vi "stimulate_pose.vi"(4 "Injection point":T4, 6 "Stimulus":sgl[](array[numeric])=[0.0, 0.0, 0.0, 0.0, 0.0, 0.0] format="%#_3p", 8 "Pose in":T1, 10 "Parameters":T2={"Stimulus"={"Type"=enum."Off", "Phase"=0.0, "Amplitude"=[], "Injection point"=enum."Total pose", "Closed loop"=FALSE, "Offset"=[], "Tip -> world"=FALSE, "Frequency"=0.0, "Length"=0.0}, "Goal Filter A"={"Speedup max"=0.0, "Speedup thresh"=0.0, "Speedup nonlin"=0.0, "Filters"=[]}, "Mode controls"={"Hold"=FALSE, "Cancellation"=FALSE, "Goal filter"=FALSE, "Trigger"=FALSE}, "Manipulator type"=enum."Current piezo", "Manipulator calibration"={"Tool offsets"=[[0.0, 0.0, 36200.0]], "Handle light calibration"=[], "Base pivots"=[], "Output pivots"=[], "Length center"=0.0, "Workspace height"=[], "Workspace diameter"=[0.0, 0.0, 36200.0], "Stack travel"=400.0, "Saturation pos"=375.0, "Inverse filters"=[], "Strut length"=0.0}, "Network"={"Remote Host"="", "Send Status"=FALSE, "Send Port"=0, "Recv Commands"=FALSE, "Recv Port"=0}, "Goal Filter B"={"Speedup max"=0.0, "Speedup thresh"=0.0, "Speedup nonlin"=0.0, "Filters"=[]}, "Cancellation"={"KP"={"XY"=0.0, "Rxy"=0.0, "Z"=0.0, "Rz"=0.0}, "KI"=0.0, "KD"={"XY"=0.0, "Rxy"=0.0, "Z"=0.0, "Rz"=0.0}, "Max vel"=20.0, "Max acc"=0.001, "Int error limit"=3.0, "RCM gain"=0.0, "Bypass"=FALSE, "Degraded gain"=0.0}, "Transition time"=0.0, "Estimation"={"Link"={"Measure noise"=[], "Process noise"=[], "Alt process noise"=[], "Alt turnoff cycles"=20, "Innovation limit"=[], "Residue threshold"=0.0, "Enable"=FALSE}, "Handle"={"Measure noise"=[], "Process noise"=[], "State limits"=[], "Innovation limit"=[], "Prediction Lookahead"=0.0, "Enable"=FALSE}}} {"Transition time" format="%_3f"; "Cancellation"."Degraded gain" min=0 max=1 step=0.1 format="%#_3p"; "Cancellation"."RCM gain" min=0 max=1 step=0.1 format="%#_3p"; "Cancellation"."KD"."Rz" min=-1 max=1 step=0.01 format="%#_3p"; "Cancellation"."KD"."Rxy" min=-1 max=1 step=0.01 format="%#_3p"; "Cancellation"."KD"."Z" min=-1 max=1 step=0.01 format="%#_3p"; "Cancellation"."KD"."XY" min=-1 max=1 step=0.01 format="%#_3p"; "Cancellation"."KI" min=0 max=1 step=0.01 format="%#_3p"; "Cancellation"."KP"."Rz" min=-1 max=1 step=0.01 format="%#_3p"; "Cancellation"."KP"."Rxy" min=-1 max=1 step=0.01 format="%#_3p"; "Cancellation"."KP"."Z" min=-1 max=1 step=0.01 format="%#_3p"; "Cancellation"."KP"."XY" min=-1 max=1 step=0.01 format="%#_3p"; "Cancellation"."Max acc" format="%#_3p"; "Goal Filter B"."Filters"."V limit range" format="%_3p"; "Goal Filter B"."Filters"."V limit" format="%_3p"; "Goal Filter B"."Filters"."Upper Q" format="%_3f"; "Goal Filter B"."Filters"."Upper Fc" format="%_3p"; "Goal Filter B"."Filters"."Lower Q" format="%_3f"; "Goal Filter B"."Filters"."Scale factor" format="%_3f"; "Goal Filter B"."Filters"."Lower Fc" format="%_3p"; "Goal Filter B"."Speedup nonlin" format="%_3p"; "Goal Filter B"."Speedup thresh" format="%_3p"; "Goal Filter B"."Speedup max" format="%_3p"; "Manipulator calibration"."Strut length" format="%#_4p"; "Manipulator calibration"."Saturation pos" format="%#.1f"; "Manipulator calibration"."Stack travel" format="%#.1f"; "Manipulator calibration"."Length center" format="%#_4p"; "Manipulator calibration"."Output pivots" format="%#_6f"; "Manipulator calibration"."Base pivots" format="%#_6f"; "Manipulator calibration"."Handle light calibration" format="%#.1f"; "Goal Filter A"."Filters"."V limit range" format="%_3p"; "Goal Filter A"."Filters"."V limit" format="%_3p"; "Goal Filter A"."Filters"."Upper Q" format="%_3f"; "Goal Filter A"."Filters"."Upper Fc" format="%_3p"; "Goal Filter A"."Filters"."Lower Q" format="%_3f"; "Goal Filter A"."Filters"."Scale factor" format="%_3f"; "Goal Filter A"."Filters"."Lower Fc" format="%_3p"; "Goal Filter A"."Speedup nonlin" format="%_3p"; "Goal Filter A"."Speedup thresh" format="%_3p"; "Goal Filter A"."Speedup max" format="%_3p"; "Stimulus"."Length" min=0.0 max=100.0 step=100.0 format="%#_4p"; "Stimulus"."Frequency" min=0.0 step=100.0 format="%#_4g"; "Stimulus"."Offset" format="%#_3p"; "Stimulus"."Amplitude" format="%#_3p"; "Stimulus"."Phase" min=-180.0 max=360.0 step=100.0 format="%#.2f"}) -> (1 "Pose out":T1)   [LabVIEW 2014]
uses:
  <vilib>/Analysis/Matrix/Datatypes/RealMatrix.ctl
  injection_point.ctl
  Micron params.ctl
  stimulus.ctl
  filtering/goal_loop_parms.ctl
  mode_conrols.ctl
  manipulator_cal.ctl
  asap/labview/testing/probe_calibration.ctl
  host/network_params.ctl
  cancellation/sq_control_params.ctl
  cancellation/decoupled_gain.ctl
  cancellation/estimation_controls.ctl
  <vilib>/Analysis/baseanly.llb/Real A x B.vi
  initialization/micron_globals.vi
  <vilib>/Analysis/Matrix/Numeric/Conversions/Array To Matrix - RA2.vi
  <vilib>/Analysis/NI_AALBase.lvlib
  <vilib>/Analysis/Matrix/NI_Matrix.lvlib
panel:
  # "Inject stimulus to pose.  Stimulus is interpreted as XYZ and Euler angles."
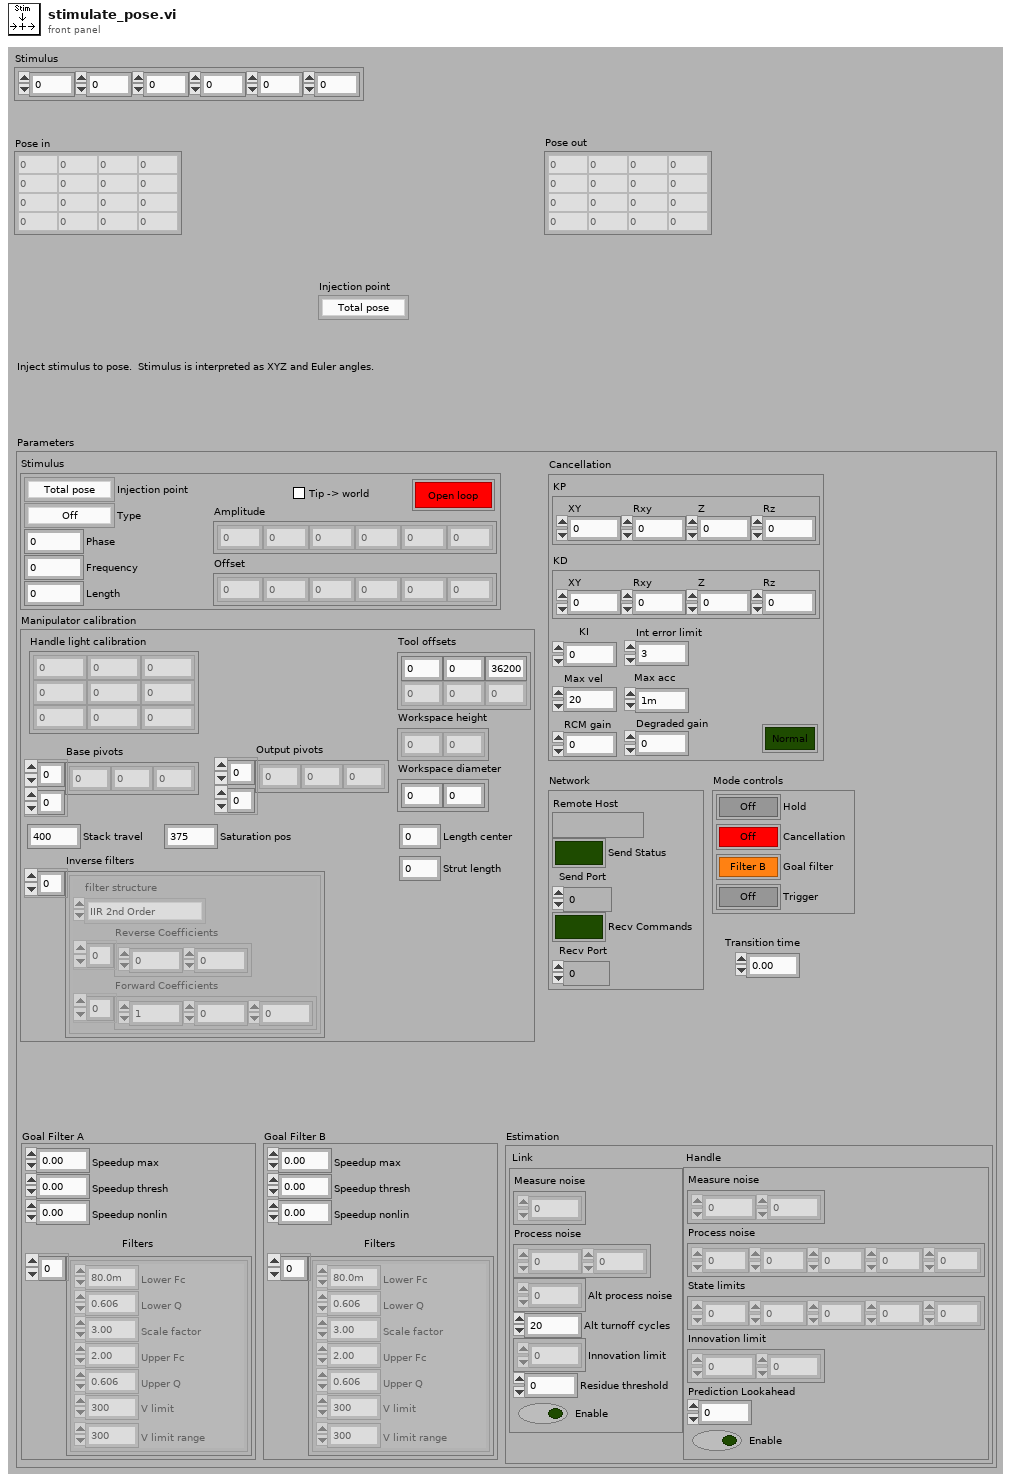
[diagram p1: front panel]
types:
  T1 = typedef "NI_Matrix.lvlib/RealMatrix.ctl" = dbl[][]
  T2 = typedef "Micron params.ctl" = cluster{"Stimulus":T3, "Goal Filter A":T5, "Mode controls":T6, "Manipulator type":enum16{"Current piezo", "Voltage piezo"}, "Manipulator calibration":T7, "Network":T9, "Goal Filter B":T5, "Cancellation":T10, "Transition time":sgl, "Estimation":T12}
  T3 = typedef "stimulus.ctl" = cluster{"Type":enum16{"Off", "Step", "Sine", "Triangle", "Arbitrary"}, "Phase":dbl, "Amplitude":sgl[], "Injection point":T4, "Closed loop":bool, "Offset":sgl[], "Tip -> world":bool, "Frequency":dbl, "Length":dbl}
  T4 = typedef "injection_point.ctl" = enum16{"Total pose", "V limiter", "Goal ", "Link position", "KF link position", "Inverse kin", "Link goal", "Link error", "Controller", "Output", "Drive", "Light"}
  T5 = typedef "goal_loop_parms.ctl" = cluster{"Speedup max":sgl, "Speedup thresh":sgl, "Speedup nonlin":sgl, "Filters":cluster{"Lower Fc":sgl, "Lower Q":sgl, "Scale factor":sgl, "Upper Fc":sgl, "Upper Q":sgl, "V limit":sgl, "V limit range":sgl}[]}
  T6 = typedef "mode_conrols.ctl" = cluster{"Hold":bool, "Cancellation":bool, "Goal filter":bool, "Trigger":bool}
  T7 = typedef "manipulator_cal.ctl" = cluster{"Tool offsets":sgl[][], "Handle light calibration":T8, "Base pivots":sgl[][], "Output pivots":sgl[][], "Length center":sgl, "Workspace height":sgl[], "Workspace diameter":sgl[], "Stack travel":sgl, "Saturation pos":sgl, "Inverse filters":cluster{"filter structure":enum32{"IIR 2nd Order", "IIR 4th Order"}, "Reverse Coefficients":dbl[], "Forward Coefficients":dbl[]}[], "Strut length":sgl}
  T8 = typedef "probe_calibration.ctl" = sgl[][]
  T9 = typedef "network_params.ctl" = cluster{"Remote Host":string, "Send Status":bool, "Send Port":u16, "Recv Commands":bool, "Recv Port":u16}
  T10 = typedef "sq_control_params.ctl" = cluster{"KP":T11, "KI":sgl, "KD":T11, "Max vel":sgl, "Max acc":sgl, "Int error limit":sgl, "RCM gain":sgl, "Bypass":bool, "Degraded gain":sgl}
  T11 = typedef "decoupled_gain.ctl" = cluster{"XY":sgl, "Rxy":sgl, "Z":sgl, "Rz":sgl}
  T12 = typedef "estimation_controls.ctl" = cluster{"Link":cluster{"Measure noise":dbl[], "Process noise":dbl[], "Alt process noise":dbl[], "Alt turnoff cycles":i32, "Innovation limit":dbl[], "Residue threshold":dbl, "Enable":bool}, "Handle":cluster{"Measure noise":dbl[], "Process noise":dbl[], "State limits":dbl[], "Innovation limit":dbl[], "Prediction Lookahead":sgl, "Enable":bool}}
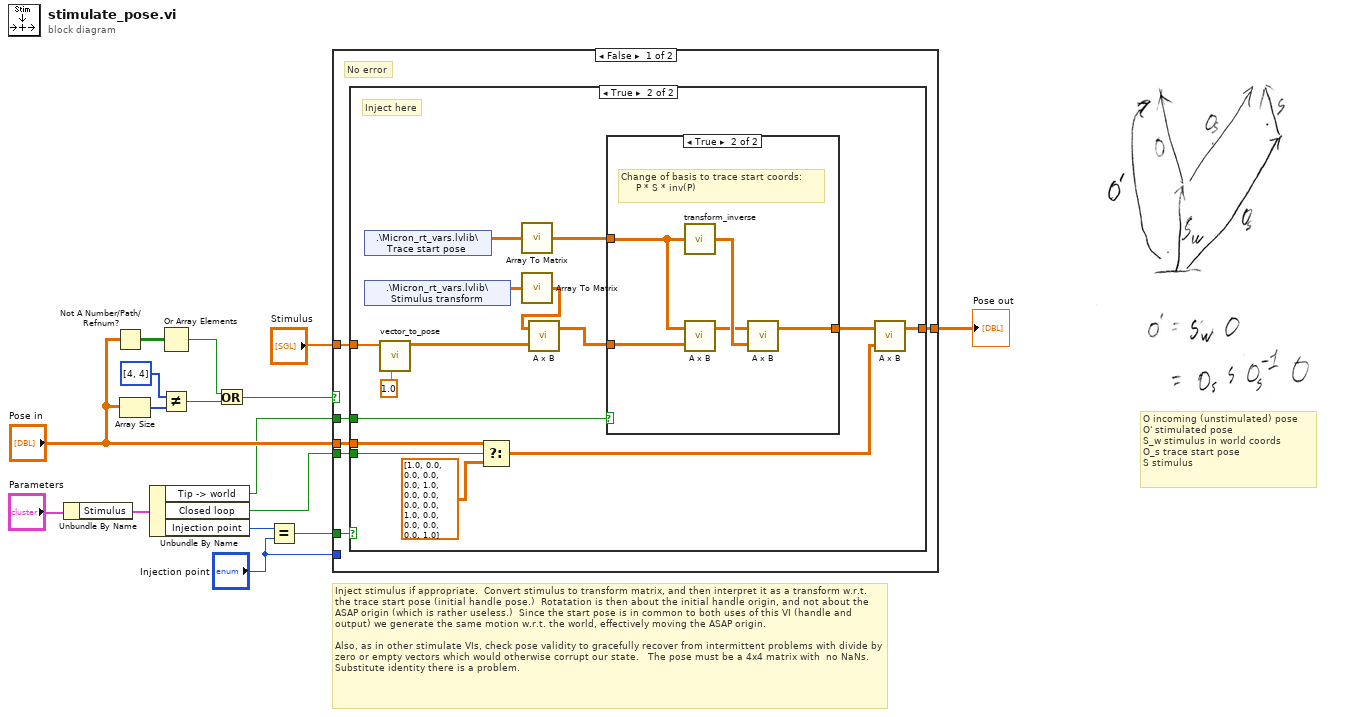
[diagram p0: block diagram]
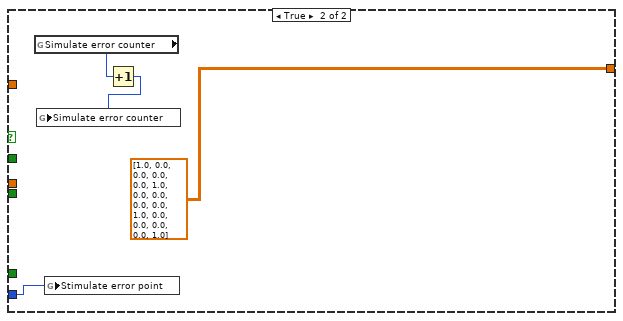
[diagram p4: hidden frame]
diagram:
  # "O incoming (unstimulated) pose\nO' stimulated pose\nS_w stimulus in world coords\nO_s trace start pose\nS stimulus"
  # "Inject stimulus if appropriate.  Convert stimulus to transform matrix, and then interpret it as a transform w.r.t. the trace start pose (initial handle pose.)  Rotatation is then about the initial handle origin, and not about the ASAP origin (which is rather useless.)  Since the start pose is in common to both uses of this VI (handle and output) we generate the same motion w.r.t. the world, effectively moving the ASAP origin.\n\nAlso, as in other stimulate VIs, check pose validity to gracefully recover from intermittent problems with divide by zero or empty vectors which would otherwise corrupt our state.   The pose must be a 4x4 matrix with  no NaNs.  Substitute identity there is a problem."
  n1 = Unbundle By Name("Parameters") -> ("Stimulus"=w10:T3)
  n2 = Not A Number/Path/Refnum?(number/path/refnum="Pose in") -> (NaN/Path/Refnum?=w8:bool[][])
  n3 = Array Size(array="Pose in") -> (size(s)=w9:i32[])
  n4 = Unbundle By Name(w10) -> ("Tip -> world"=w1:bool, "Closed loop"=w14:bool, "Injection point"=w12:T4)
  n5 = Or Array Elements(Boolean array=w8) -> (logical OR=w7:bool)
  n6 = Not Equal?(x=i32[] [4, 4], y=w9) -> (x != y?=w6:bool)
  n7 = Or(x=w7, y=w6) -> (x .or. y?=w5:bool)
  n8 = Equal?(x=w12, y="Injection point") -> (x = y?=w16:bool)
  n9 = case shown="False" w5 {
    tunnel: w16 -> [w22 _]
    tunnel: "Pose in" -> [w21 _]
    tunnel: [w20 sgl[][] [[1.0, 0.0, 0.0, 0.0], [0.0, 1.0, 0.0, 0.0], [0.0, 0.0, 1.0, 0.0], [0.0, 0.0, 0.0, 1.0]] ("Stimulus")] -> w15
    tunnel: w14 -> [w19 _]
    tunnel: "Stimulus" -> [w18 _]
    tunnel: "Injection point" -> [_ w45]
    tunnel: w1 -> [w17 _]
    frame False {
      # "No error"
      n10 = case shown="True" w22 {
        tunnel: w21 -> [w23 w31]
        tunnel: w18 -> [_ w38]
        tunnel: [w23 w24] -> w20
        tunnel: w19 -> [_ w32]
        tunnel: w17 -> [_ w36]
        frame False {
          # "No injection here"
        }
        frame True {
          # "Inject here"
          n11 = shared-variable ".\\Micron_rt_vars.lvlib\\Trace start pose"() -> (w28:sgl[][])  [unwired: 2 out]
          n12 = shared-variable ".\\Micron_rt_vars.lvlib\\Stimulus transform"() -> (w34:sgl[][])  [unwired: 2 out]
          n13 = call "vector_to_pose.vi"("Translation scale"=1.0, "Pose vector"=w38) -> ("Pose"=w35:T1)  [unwired: 9 in]
          n14 = Select(t=w31, s=w32, f=T1 [[1.0, 0.0, 0.0, 0.0], [0.0, 1.0, 0.0, 0.0], [0.0, 0.0, 1.0, 0.0], [0.0, 0.0, 0.0, 1.0]] ("Pose")) -> (s? t:f=w26:T1)
          n15 = call-poly <vilib>:"Array To Matrix.vi"("Real 2D Array"=w28) -> ("Real Matrix"=w27:T1)
          n16 = call-poly <vilib>:"Array To Matrix.vi"("Real 2D Array"=w34) -> ("Real Matrix"=w33:T1)
          n17 = call-poly <vilib>:"A x B.vi"("B"=w35, "A"=w33) -> ("A x B"=w29:T1)  [unwired: 1 out]
          n18 = case shown="True" w36 {
            tunnel: w29 -> [w39 w41]
            tunnel: [w39 w42] -> w25
            tunnel: w27 -> [_ w40]
            frame False {
              # "No transform"
            }
            frame True {
              # "Change of basis to trace start coords:\n     P * S * inv(P)"
              n19 = call "transform_inverse.vi"("Transform"=w40) -> ("Inverse transform"=w44:T1)
              n20 = call-poly <vilib>:"A x B.vi"("B"=w41, "A"=w40) -> ("A x B"=w43:T1)  [unwired: 1 out]
              n21 = call-poly <vilib>:"A x B.vi"("B"=w44, "A"=w43) -> ("A x B"=w42:T1)  [unwired: 1 out]
            }
          }
          n22 = call-poly <vilib>:"A x B.vi"("B"=w26, "A"=w25) -> ("A x B"=w24:T1)  [unwired: 1 out]
        }
      }
    }
    frame True {
      n23 = global read "micron_globals.vi" "Simulate error counter"() -> (w47:i32)
      n24 = global write "micron_globals.vi" "Stimulate error point"(w45) -> ()
      n25 = Increment(x=w47) -> (x+1=w46:i32)
      n26 = global write "micron_globals.vi" "Simulate error counter"(w46) -> ()
    }
  }
  "Pose out" <- w15
